vi "LinkNodes.vi"(6 "index":i32, 8 "error in":errorcluster, 10 "child in":T1, 11 "parent in":T1) -> (0 "error out":errorcluster, 2 "child out":T1, 3 "parent out":T1)   [LabVIEW 2023, in "CEF.lvlib" / "CEF_Node.lvclass"]
doc: "Links 2 nodes together one as a parent and one as a child.Copyright 2017 National Instruments Corporation\n\nLicensed under the Apache License, Version 2.0 (the \"License\"); you may not use this file except in compliance with the License. You may obtain a copy of the License at http://www.apache.org/licenses/LICENSE-2.0\nUnless required by applicable law or agreed to in writing, software distributed under the License is distributed on an \"AS IS\" BASIS, WITHOUT WARRANTIES OR CONDITIONS OF ANY KIND, either express or implied. See the License for the specific language governing permissions and limitations under the License."
uses:
  CEF_Node.lvclass
  NodeRef.ctl
  CEF_Node.lvclass/CEF_Node.ctl
  ReadChildren.vi
  WriteChildren.vi
  WriteParent.vi
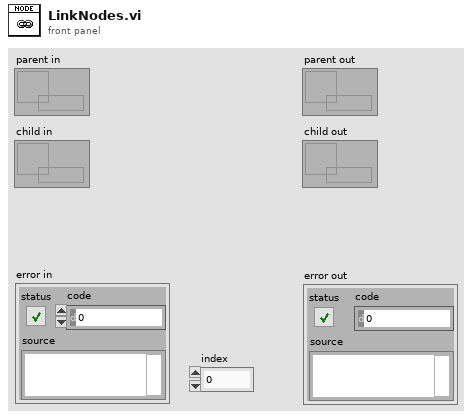
[diagram p1: front panel]
types:
  T1 = typedef "CEF.lvlib/CEF_Node.lvclass/NodeRef.ctl" = refnum<data-value>
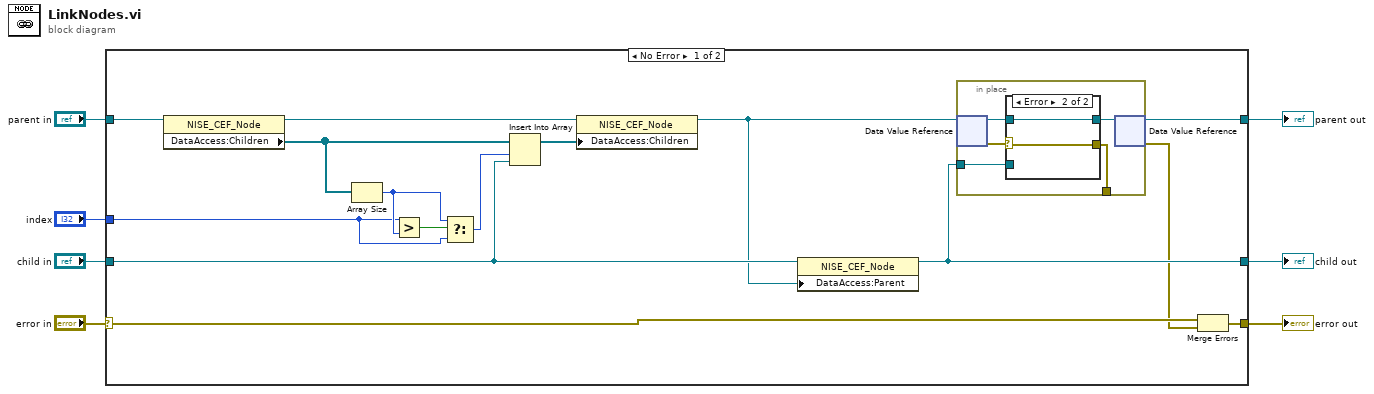
[diagram p0: block diagram]
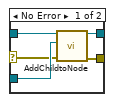
[diagram p2: hidden frame]
diagram:
  n1 = case shown="No Error" "error in" {
    selector: "error in" -> [w22 w37]
    tunnel: [w10 w37] -> w3
    tunnel: "parent in" -> [w16 w36]
    tunnel: "child in" -> [w14 w35]
    tunnel: [w12 w35] -> w2
    tunnel: [w11 w36] -> w1
    tunnel: "index" -> [w19 _]
    frame No Error {
      n2 = property class="NISE_CEF_Node"(reference=w16) -> (reference out=w15:T1, "DataAccess:Children"=w18:T1[])  [unwired: 1 in, 1 out]
      n3 = Array Size(array=w18) -> (size(s)=w20:i32)
      n4 = Greater?(x=w19, y=w20) -> (0:w21:bool)
      n5 = Select(t=w20, s=w21, f=w19) -> (s? t:f=w17:i32)
      n6 = Insert Into Array(array=w18, index=w17, new element=w14) -> (w8:T1[])
      n7 = property class="NISE_CEF_Node"(reference=w15, "DataAccess:Children"=w8) -> (reference out=w13:T1)  [unwired: 1 in, 1 out]
      n8 = property class="NISE_CEF_Node"(reference=w14, "DataAccess:Parent"=w13) -> (reference out=w12:T1)  [unwired: 1 in, 1 out]
      n9 = in-place {
        in-place-border: w12 -> [w24]
        in-place-border: [w23] -> _
        n10 = in-place-dvr #1(w13) -> (w27:refnum<class "CEF_Node.lvclass">, w25:errorcluster)
        n11 = case shown="Error" w25 {
          selector: w25 -> [w28 w33]
          tunnel: w27 -> [w32 w34]
          tunnel: [w31 w34] -> w26
          tunnel: [w30 w33] -> w23
          tunnel: w24 -> [w29 _]
          frame No Error {
            n12 = call-dynamic "AddChildtoNode.vi"("error in"=w28, "child in"=w29, "CEF_Node in"=w32) -> ("error out"=w30:errorcluster, "CEF_Node out"=w31:refnum<class "CEF_Node.lvclass">)  [unwired: 7 in]
          }
          frame Error {
          }
        }
        n13 = in-place-dvr #1(w26) -> (w11:T1, w9:errorcluster)
      }
      n14 = Merge Errors(w22, w9) -> (w10:errorcluster)
    }
    frame Error {
    }
  }
  "error out" <- w3
  "child out" <- w2
  "parent out" <- w1
